vi "Get Thermal Information.vi"(8 "error in":errorcluster, 11 "All Data":T1 {"PLC Data"."PLC Data - LDO"."Timing"."Absolute Time" format="%<%H:%M:%S%3u>t"; "PLC Data"."PLC Data - LDO"."Timing"."Display Time" format="%#.20f"; "PLC Data"."PLC Data - LDO"."Timing"."Test Time Ref" format="%#.20f"; "PLC Data"."PLC Data - LDO"."Timing"."Precondition Time Ref" format="%#.20f"; "PLC Data"."PLC Data - LDO"."Timing"."First Call Time Ref" format="%#.20f"; "PLC Data"."PLC Data - FVIR"."Timing"."Absolute Time" format="%<%H:%M:%S%3u>t"; "PLC Data"."PLC Data - FVIR"."Timing"."Display Time" format="%#.20f"; "PLC Data"."PLC Data - FVIR"."Timing"."Test Time Ref" format="%#.20f"; "PLC Data"."PLC Data - FVIR"."Timing"."Precondition Time Ref" format="%#.20f"; "PLC Data"."PLC Data - FVIR"."Timing"."First Call Time Ref" format="%#.20f"}) -> (0 "error out":errorcluster, 3 "All Data Out":T1 {"PLC Data"."PLC Data - LDO"."Timing"."Absolute Time" format="%<%H:%M:%S%3u>t"; "PLC Data"."PLC Data - LDO"."Timing"."Display Time" format="%#.20f"; "PLC Data"."PLC Data - LDO"."Timing"."Test Time Ref" format="%#.20f"; "PLC Data"."PLC Data - LDO"."Timing"."Precondition Time Ref" format="%#.20f"; "PLC Data"."PLC Data - LDO"."Timing"."First Call Time Ref" format="%#.20f"; "PLC Data"."PLC Data - FVIR"."Timing"."Absolute Time" format="%<%H:%M:%S%3u>t"; "PLC Data"."PLC Data - FVIR"."Timing"."Display Time" format="%#.20f"; "PLC Data"."PLC Data - FVIR"."Timing"."Test Time Ref" format="%#.20f"; "PLC Data"."PLC Data - FVIR"."Timing"."Precondition Time Ref" format="%#.20f"; "PLC Data"."PLC Data - FVIR"."Timing"."First Call Time Ref" format="%#.20f"})   [LabVIEW 2020]
uses:
  Modbus/Modbus All Data.ctl
  Modbus/Modbus PLC Data All.ctl
  Modbus/Modbus FVIR Control.ctl
  Modbus/Modbus Timing.ctl
  <vilib>/Utility/miscctls.llb/LVDateTimeRec.ctl
  Modbus/Modbus LDO Control.ctl
  WritingDataFile/Data to Save.ctl
  Terminate Conditions Cluster.ctl
  Drivers/Inficon Transmitter/Type Definitions/Inficon Data.ctl
  Modbus/Modbus Gas Meter Data.ctl
  Drivers/Alicat LabVIEW Drivers 2v1/Sub-VIs/Data Cluster.ctl
  Drivers/Alicat LabVIEW Drivers 2v1/Sub-VIs/Units of Measure.ctl
  Gas_Rate/HEWH ANSI Rate.ctl
  Drivers/Resideo Gas Valve/Type Definitions/Vesta Info.ctl
  Thermal Calculation Cluster.ctl
panel:
  in  "LDO Full Data-Debug":string[][](array[string])=[["System Date", "06/23/2022"], ["System Time", "11:21:28.543"], ["Elapsed Time (sec)", "35"], ["PLC Real-Time Clock (Min)", "0.600000"], ["Water Inlet - Temperature (°F) - PL0001", "69.010000"], ["Water Outlet - Temperature (°F) - PL0002", "69.300000"], ["Ambient Temperature (°F)- PL0003", "68.760000"], ["Flue Exhaust Collector Box Top(°F)- PL0004", "68.970000"], ["Cold Supply Temperature (°F)- PL0005", "69.970000"], ["Hot Supply Temperature (°F)- PL0006", "68.960000"], ["TC Down (°F)- PL0007", "69.220000"], ["Ambient Temperature Outside Chamber (°F)- PL0008", "70.120000"], ["Flue Exhaust Collector Elbow (°F)- PL0009", "69.260000"], ["LDO Room Ceiling (°F)- PL0010", "69.510000"], ["Flue Gas Temperature (°F) - PL0011", "69.670000"], ["TC Type J (°F) - PL0012", "2187.000000"], ["TC Type J (°F) - PL0013", "2187.000000"], ["TC Type J (°F) - PL0014", "2187.000000"], ["TC Type K (°F) - PL0015", "2496.600000"], ["TC Type K (°F) - PL0016", "2496.600000"], ["TC Type K (°F)- PL0017", "2496.600000"], ["TC Type K (°F)- PL0018", "2496.600000"], ["Pilot Millivoltage (mV)", "0.000000"], ["Room Differential Pressure (in Water)", "0.002000"], ["Gas Manifold Pressure (in Water)", "0.120000"], ["Water Pressure Sensor (PSI)", "0.000000"], ["Flow Rate (GPM)", "0.000000"], ["Totalized Flow (Gallons)", "0.000000"], ["Counter of oil injections 0.8 cc/min", "1.000000"], ["Counter of oil injections 1.1 cc/min", "1.000000"], ["Counter of oil injections 1.33 cc/min", "13.000000"], ["Total Cycle Counter", "13.000000"], ["Absolute Pressure [inHgA]", "28.290000"], ["Gauge/Diff. Pressure [inHgG]", "-1.150000"], ["BarometricPressure [inHgA]", "29.434000"], ["Temperature [°F]", "72.800000"], ["Uncorrected [CFH]", "-0.324000"], ["Corrected [SCFH]", "-0.298000"], ["Gas Rate (BTU/hr)", "-318.821368"], ["Energy (BTU)", "0.000000"], ["Heating Value (BTU/cu.ft)", "1069.870361"], ["Totalizer [Sft3]", "0.000000"], ["Gas Selected", "NatG-1"], ["Channel Status", "Measure"], ["CO(PPMv)", "34.000"], ["CO2(%)", "0.000"], ["O2(%)", "20.890"], ["CO2 Air Free-Ultimate (%)\t\t\t\t\t\t\t\t\t", "12.200"], ["Air Free Factor", "Inf"], ["CO Air Free (%)", "Inf"], ["Water Outlet Valve-LDO", "0"], ["Water Inlet Valve-LDO", "0"], ["Gas Solenoid Valve-LDO", "1"], ["Water Flow DRK375-LDO", "0"], ["Oil Spray 0.8 cc/min-LDO", "0"], ["Oil Spray 1.1 cc/min-LDO", "0"], ["Oil Spray 1.33 cc/min-LDO", "0"], ["Heater ON/OFF-LDO", "0"], ["Water Outlet Proportional Valve-LDO", "0"], ["Conveyor ON/OFF", "0"], ["Blower ON/OFF", "0"], ["Reset LDO Totalizer (Status)", "0"]]
  # "Totalizer Timer"
  # "Totalizer Timer"
  # "Natural Gas"
  # "Propane"
  # "Totalizer Timer"
  # "Totalizer Timer"
  # "Natural Gas"
  # "Propane"
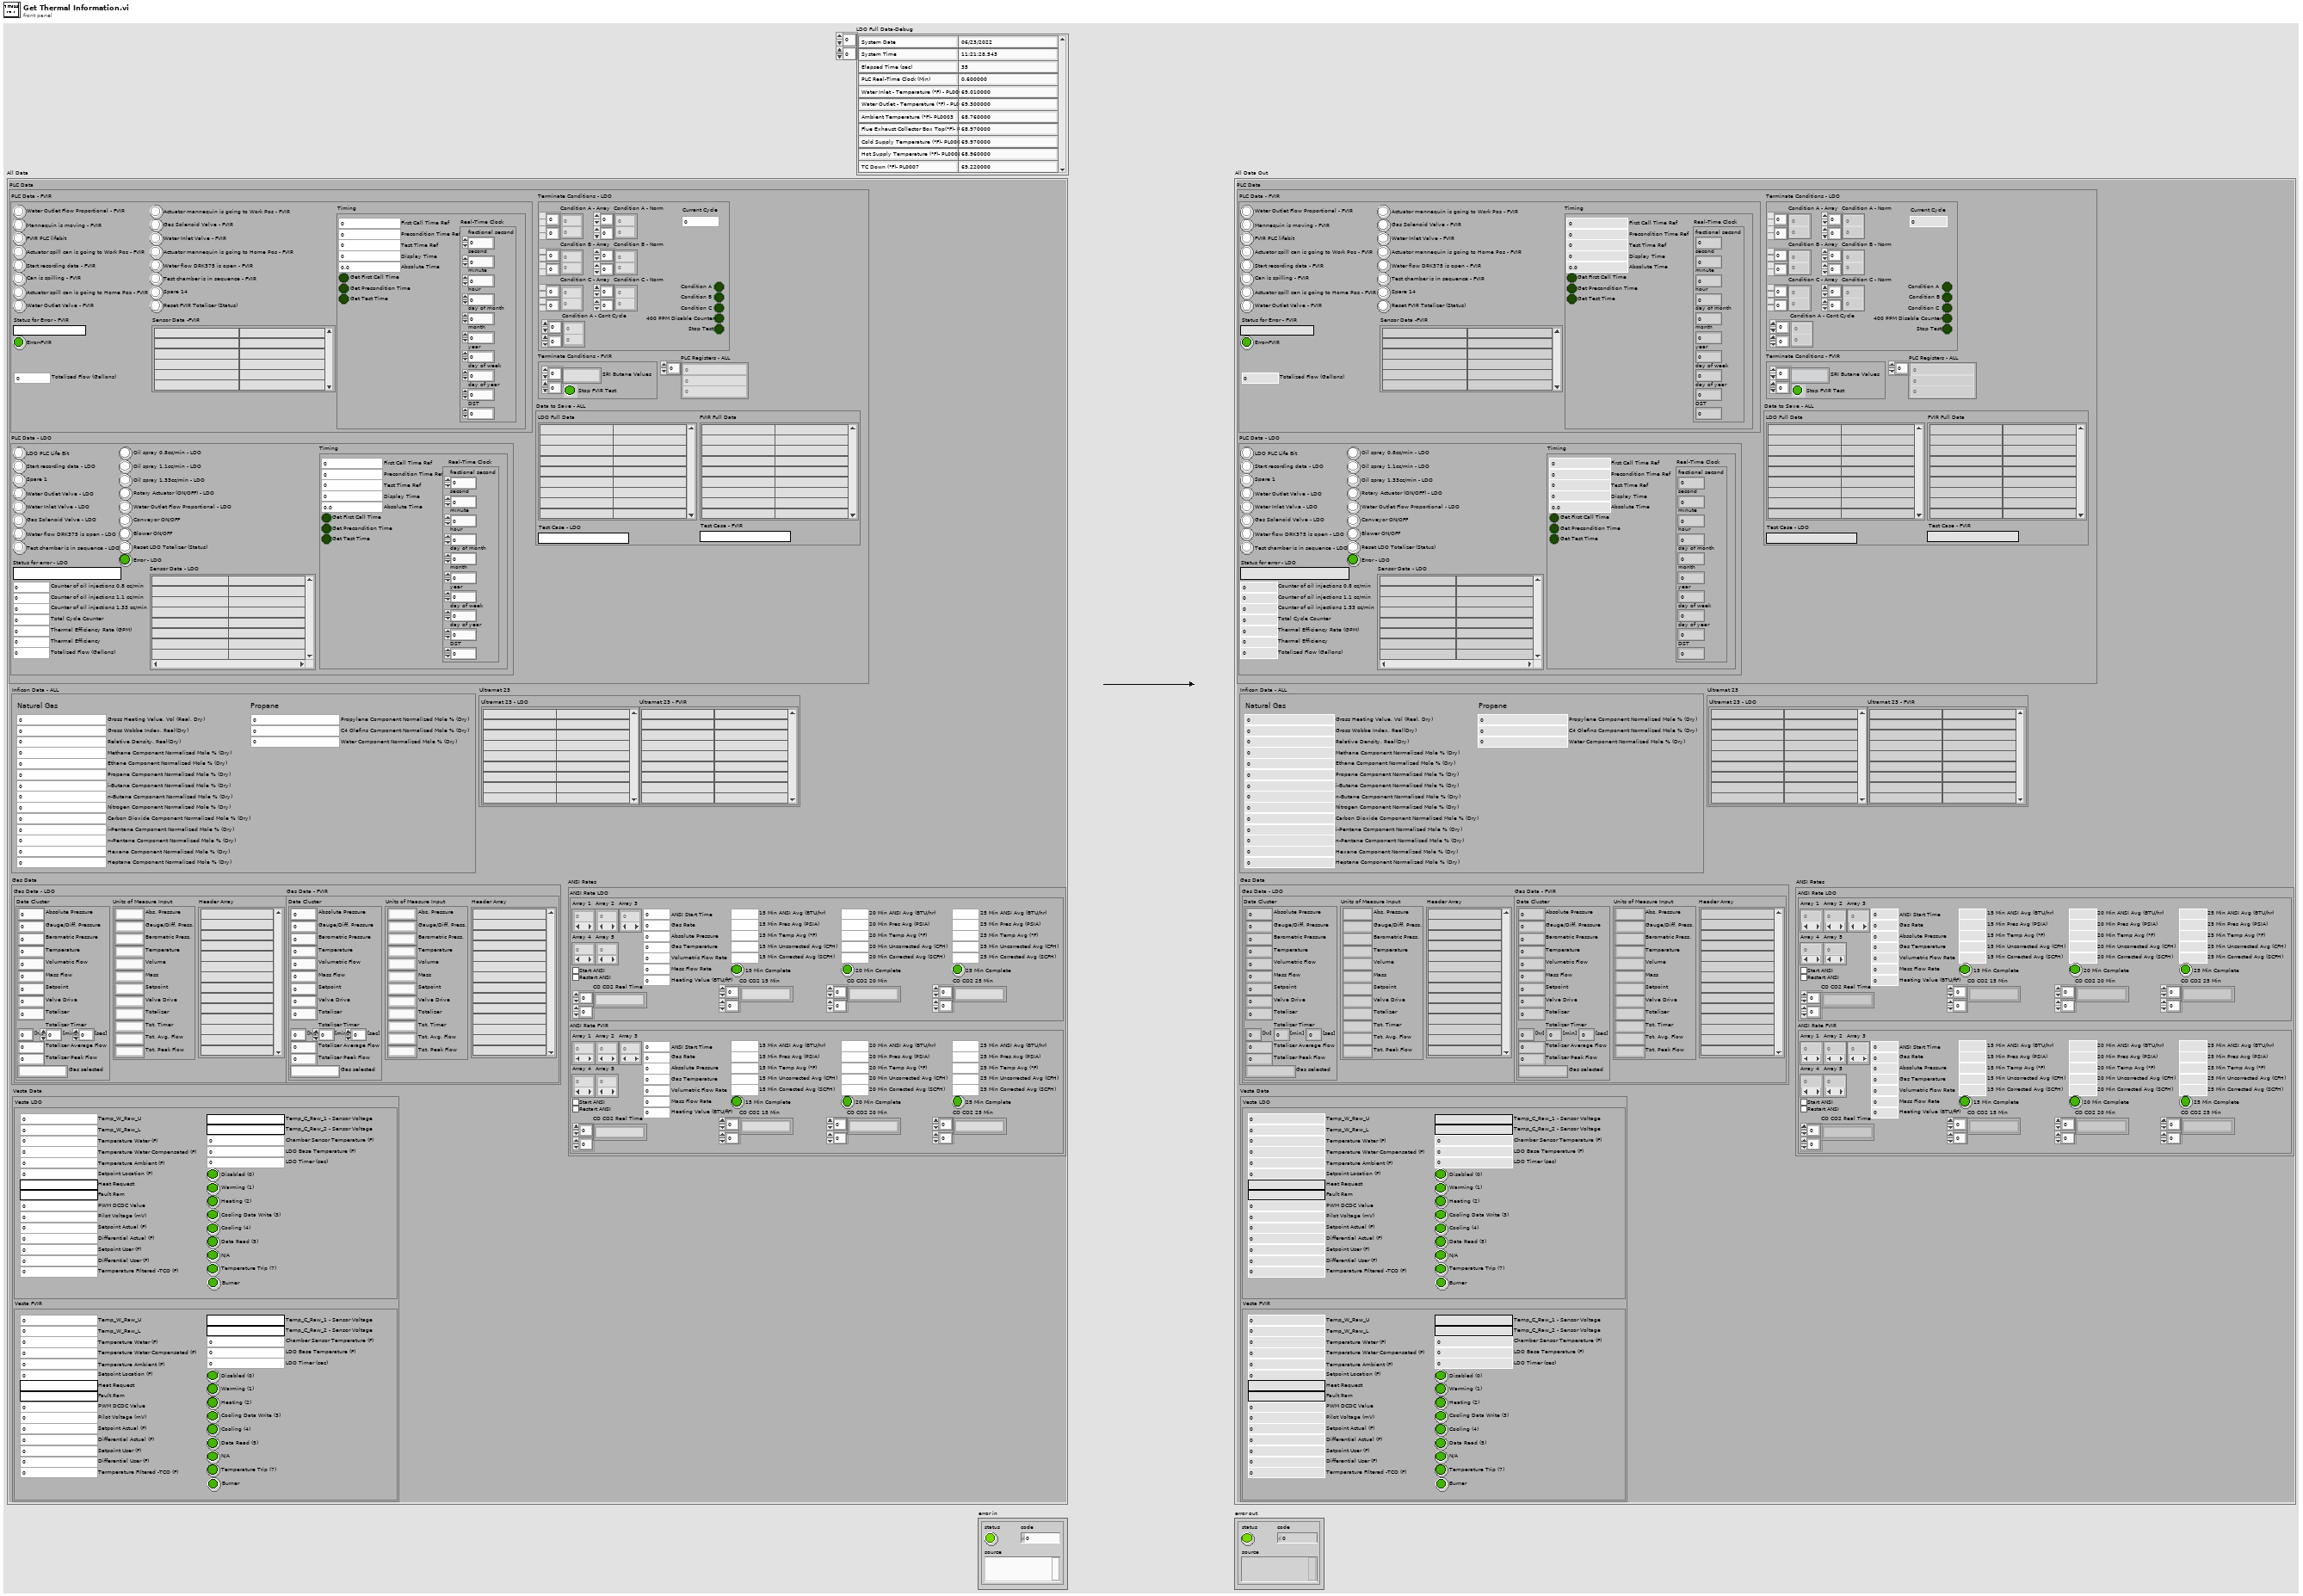
[diagram p1: front panel]
types:
  T1 = typedef "Modbus All Data.ctl" = cluster{"PLC Data":T2, "Inficon Data - ALL":T9, "Gas Data":cluster{"Gas Data - LDO":T10, "Gas Data - FVIR":T10}, "Ultramat 23":cluster{"Ultramat 23 - LDO":string[][], "Ultramat 23 - FVIR":string[][]}, "ANSI Rates":cluster{"ANSI Rate LDO":T13, "ANSI Rate FVIR":T13}, "Vesta Data":cluster{"Vesta LDO":T14, "Vesta FVIR":T14}}
  T2 = typedef "Modbus PLC Data All.ctl" = cluster{"PLC Data - FVIR":T3, "PLC Data - LDO":T6, "PLC Registers - ALL":i16[], "Data to Save - ALL":T7, "Terminate Conditions - LDO":T8, "Terminate Conditions - FVIR":cluster{"SRI Butane Values":string[][], "Stop FVIR Test":bool}}
  T3 = typedef "Modbus FVIR Control.ctl" = cluster{"Reset FVIR Totalizer (Status)":bool, "Spare 14":bool, "Actuator mannequin is going to Work Pos - FVIR":bool, "Actuator mannequin is going to Home Pos - FVIR":bool, "Test chamber is in sequence - FVIR ":bool, "Water flow DRK375 is open - FVIR":bool, "Gas Solenoid Valve - FVIR":bool, "Water Inlet Valve - FVIR":bool, "Water Outlet Flow Proportional - FVIR":bool, "Start recording data - FVIR":bool, "Actuator spill can is going to Work Pos - FVIR":bool, "Actuator spill can is going to Home Pos - FVIR":bool, "Water Outlet Valve - FVIR":bool, "Can is spilling - FVIR":bool, "Mannequin is moving - FVIR":bool, "FVIR PLC lifebit":bool, "Status for Error - FVIR":string, "Error-FVIR":bool, "Sensor Data -FVIR":string[][], "Totalized Flow (Gallons)":dbl, "Timing":T4}
  T4 = typedef "Modbus Timing.ctl" = cluster{"First Call Time Ref":dbl, "Precondition Time Ref":dbl, "Test Time Ref":dbl, "Get First Call Time":bool, "Get Precondition Time":bool, "Get Test Time":bool, "Display Time":dbl, "Real-Time Clock":T5, "Absolute Time":dbl}
  T5 = typedef "LVDateTimeRec.ctl" = cluster{"fractional second":dbl, "second":i32, "minute":i32, "hour":i32, "day of month":i32, "month":i32, "year":i32, "day of week":i32, "day of year":i32, "DST":i32}
  T6 = typedef "Modbus LDO Control.ctl" = cluster{"LDO PLC Life Bit":bool, "Start recording data - LDO":bool, "Spare 1":bool, "Water Outlet Valve - LDO":bool, "Water Inlet Valve - LDO":bool, "Gas Solenoid Valve - LDO":bool, "Water flow DRK375 is open - LDO":bool, "Test chamber is in sequence - LDO":bool, "Oil spray 0.8cc/min - LDO":bool, "Oil spray 1.1cc/min - LDO":bool, "Oil spray 1.33cc/min - LDO":bool, "Rotary Actuator (ON/OFF) - LDO":bool, "Water Outlet Flow Proportional - LDO":bool, "Conveyor ON/OFF":bool, "Blower ON/OFF":bool, "Reset LDO Totalizer (Status)":bool, "Status for error - LDO":string, "Error - LDO":bool, "Sensor Data - LDO":string[][], "Thermal Efficiency Rate (GPM)":dbl, "Thermal Efficiency":dbl, "Totalized Flow (Gallons)":dbl, "Counter of oil injections 1.33 cc/min":u16, "Total Cycle Counter":u16, "Counter of oil injections 1.1 cc/min":u16, "Counter of oil injections 0.8 cc/min":u16, "Timing":T4}
  T7 = typedef "Data to Save.ctl" = cluster{"LDO Full Data":string[][], "FVIR Full Data":string[][], "Test Case - FVIR":string, "Test Case - LDO":string}
  T8 = typedef "Terminate Conditions Cluster.ctl" = cluster{"Condition B - Array":dbl[][], "Current Cycle":u16, "Condition C - Array":dbl[][], "Condition A - Array":dbl[][], "400 PPM Disable Counter":bool, "Condition A - Norm":dbl[][], "Condition B - Norm":dbl[][], "Condition C - Norm":dbl[][], "Condition A":bool, "Condition B":bool, "Condition C":bool, "Condition A - Cont Cycle":dbl[][], "Stop Test":bool}
  T9 = typedef "Inficon Data.ctl" = cluster{"Gross Heating Value, Vol (Real, Dry)":dbl, "Nitrogen Component Normalized Mole % (Dry)":dbl, "Methane Component Normalized Mole % (Dry)":dbl, "Carbon Dioxide Component Normalized Mole % (Dry)":dbl, "Ethane Component Normalized Mole % (Dry)":dbl, "Propane Component Normalized Mole % (Dry)":dbl, "i-Pentane Component Normalized Mole % (Dry)":dbl, "i-Butane Component Normalized Mole % (Dry)":dbl, "n-Butane Component Normalized Mole % (Dry)":dbl, "n-Pentane Component Normalized Mole % (Dry)":dbl, "Hexane Component Normalized Mole % (Dry)":dbl, "Heptane Component Normalized Mole % (Dry)":dbl, "Gross Wobbe Index, Real(Dry)":dbl, "Relative Density, Real(Dry)":dbl, "Propylene Component Normalized Mole % (Dry)":dbl, "C4 Olefins Component Normalized Mole % (Dry)":dbl, "Water Component Normalized Mole % (Dry)":dbl}
  T10 = typedef "Modbus Gas Meter Data.ctl" = cluster{"Data Cluster":T11, "Units of Measure Input":T12, "Header Array":string[]}
  T11 = typedef "Data Cluster.ctl" = cluster{"Absolute Pressure":dbl, "Gauge/Diff. Pressure":dbl, "Barometric Pressure":dbl, "Temperature":dbl, "Volumetric Flow":dbl, "Mass Flow":dbl, "Setpoint":dbl, "Valve Drive":dbl, "Totalizer":dbl, "[hr]":dbl, "[min]":dbl, "[sec]":dbl, "Totalizer Average Flow":dbl, "Totalizer Peak Flow":dbl, "Gas selected":string}
  T12 = typedef "Units of Measure.ctl" = cluster{"Abs. Pressure":string, "Gauge/Diff. Press.":string, "Barometric Press.":string, "Temperature":string, "Volume":string, "Mass":string, "Setpoint":string, "Valve Drive":string, "Totalizer":string, "Tot. Timer":string, "Tot. Avg. Flow":string, "Tot. Peak Flow":string}
  T13 = typedef "HEWH ANSI Rate.ctl" = cluster{"Array 1":dbl[], "Array 3":dbl[], "Array 2":dbl[], "Start ANSI":bool, "ANSI Start Time":dbl, "Restart ANSI":bool, "15 Min ANSI Avg (BTU/hr)":dbl, "20 Min ANSI Avg (BTU/hr)":dbl, "25 Min ANSI Avg (BTU/hr)":dbl, "Absolute Pressure":dbl, "Gas Temperature":dbl, "Volumetric Flow Rate":dbl, "Mass Flow Rate":dbl, "Array 4":dbl[], "Array 5":dbl[], "Gas Rate":dbl, "15 Min Pres Avg (PSIA)":dbl, "20 Min Pres Avg (PSIA)":dbl, "25 Min Pres Avg (PSIA)":dbl, "15 Min Temp Avg (°F) ":dbl, "20 Min Temp Avg (°F)":dbl, "25 Min Temp Avg (°F)":dbl, "15 Min Uncorrected Avg (CFH)":dbl, "20 Min Uncorrected Avg (CFH)":dbl, "25 Min Uncorrected Avg (CFH)":dbl, "15 Min Corrected Avg (SCFH)":dbl, "20 Min Corrected Avg (SCFH)":dbl, "25 Min Corrected Avg (SCFH)":dbl, "15 Min Complete":bool, "20 Min Complete":bool, "25 Min Complete":bool, "Heating Value (BTU/ft³)":dbl, "CO CO2 15 Min":string[][], "CO CO2 20 Min":string[][], "CO CO2 25 Min":string[][], "CO CO2 Real Time":string[][]}
  T14 = typedef "Vesta Info.ctl" = cluster{"Temp_W_Raw_U":u16, "Temp_W_Raw_L":u16, "Temperature Water (F)":dbl, "Temperature Water Compensated (F)":dbl, "Temperature Ambient (F)":dbl, "Setpoint Location (F)":dbl, "Heat Request":string, "Fault Ram":string, "PWM DCDC Value":u16, "Pilot Voltage (mV)":dbl, "Setpoint Actual (F)":dbl, "Differential Actual (F)":dbl, "Setpoint User (F)":dbl, "Differential User (F)":dbl, "Termperature FIltered -TCO (F)":dbl, "Temp_C_Raw_1 - Sensor Voltage":string, "Temp_C_Raw_2 - Sensor Voltage":string, "Chamber Sensor Temperature (F)":dbl, "LDO Base Temperature (F)":dbl, "LDO Timer (sec)":i16, "Disabled (0)":bool, "Warming (1)":bool, "Heating (2)":bool, "Cooling Data Write (3)":bool, "Cooling (4)":bool, "Data Read (5)":bool, "N/A":bool, "Temperature Trip (7)":bool, "Burner":bool}
  T15 = typedef "Thermal Calculation Cluster.ctl" = cluster{"Gross Heating Value, Vol (Real, Dry)":dbl, "RTD Out (Deg F)":dbl, "RTD In (Deg F)":dbl, "Gallons (Gal)":dbl, "Gas Mass Flow":dbl, "Gas Totalizer":dbl, "Use Constant Thermal Efficiency":bool, "Constant Thermal Eff":dbl}
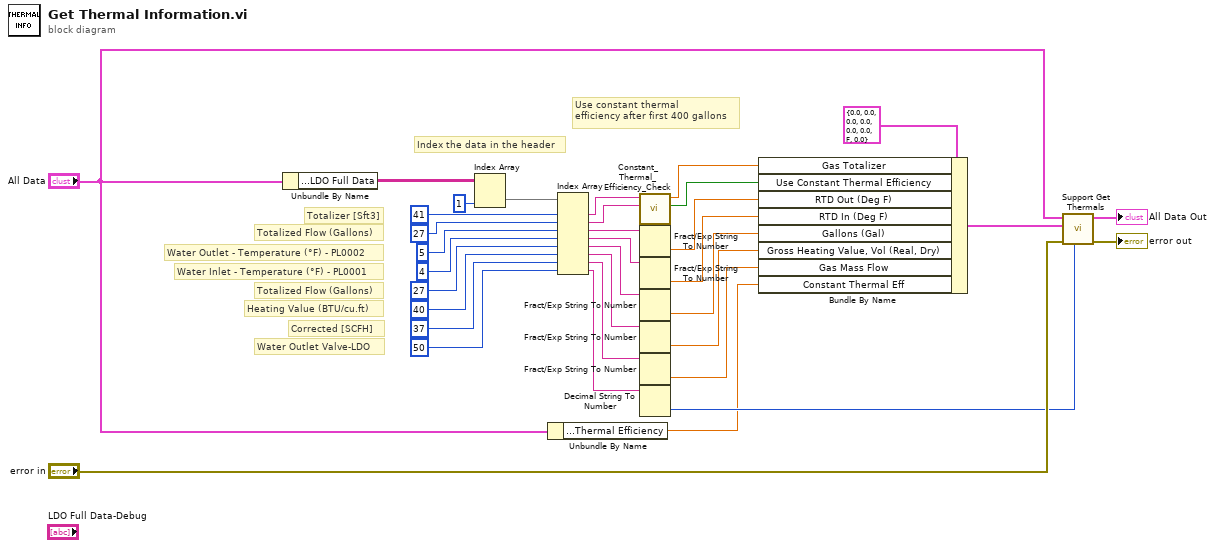
[diagram p0: block diagram]
diagram:
  # "Use constant thermal\nefficiency after first 400 gallons"
  # "Water Outlet Valve-LDO"
  # "Totalized Flow (Gallons)"
  # "Totalizer [Sft3]"
  # "Corrected [SCFH]"
  # "Heating Value (BTU/cu.ft)"
  # "Totalized Flow (Gallons)"
  # "Water Outlet - Temperature (°F) - PL0002"
  # "Water Inlet - Temperature (°F) - PL0001"
  # "Index the data in the header"
  n1 = Unbundle By Name("All Data") -> ("PLC Data.Data to Save - ALL.LDO Full Data"=w10:string[][])
  n2 = Index Array(array=w10, index (col)=1 ("disabled index (col)")) -> (element=w27:string[])  [unwired: 1 in]
  n3 = Unbundle By Name("All Data") -> ("PLC Data.PLC Data - LDO.Thermal Efficiency"=w1:dbl)
  n4 = Index Array(array=w27, index #1=41 ("index"), index #2=27 ("index"), index #3=5 ("index"), index #4=4 ("index"), index #5=27 ("index"), index #6=40 ("index"), index #7=37 ("index"), index #8=50 ("index")) -> (element #1=w26:string, element #2=w11:string, element #3=w17:string, element #4=w16:string, element #5=w15:string, element #6=w14:string, element #7=w13:string, element #8=w12:string)
  n5 = call "Constant_Thermal_Efficiency_Check.vi"("Totalized Flow (Gallons)"=w11, "Totalizer [Sft3]"=w26) -> ("Constant Thermal Efficiency?"=w7:bool, "Totalizer [Sft3]"=w8:dbl)  [unwired: 8 in]
  n6 = Fract/Exp String To Number(string=w17) -> (number=w6:dbl)  [unwired: 3 in, 1 out]
  n7 = Fract/Exp String To Number(string=w16) -> (number=w5:dbl)  [unwired: 3 in, 1 out]
  n8 = Fract/Exp String To Number(string=w15) -> (number=w4:dbl)  [unwired: 3 in, 1 out]
  n9 = Fract/Exp String To Number(string=w14) -> (number=w3:dbl)  [unwired: 3 in, 1 out]
  n10 = Fract/Exp String To Number(string=w13) -> (number=w2:dbl)  [unwired: 3 in, 1 out]
  n11 = Decimal String To Number(string=w12) -> (number=w31:i32)  [unwired: 2 in, 1 out]
  n12 = Bundle By Name(cluster=T15 {"Gross Heating Value, Vol (Real, Dry)"=0.0, "RTD Out (Deg F)"=0.0, "RTD In (Deg F)"=0.0, "Gallons (Gal)"=0.0, "Gas Mass Flow"=0.0, "Gas Totalizer"=0.0, "Use Constant Thermal Efficiency"=FALSE, "Constant Thermal Eff"=0.0} ("Input Data"), "Gas Totalizer"=w8, "Use Constant Thermal Efficiency"=w7, "RTD Out (Deg F)"=w6, "RTD In (Deg F)"=w5, "Gallons (Gal)"=w4, "Gross Heating Value, Vol (Real, Dry)"=w3, "Gas Mass Flow"=w2, "Constant Thermal Eff"=w1) -> (w29:T15)
  n13 = call "Support Get Thermals.vi"("Water Outlet Valve"=w31, "error in"="error in", "Input Data"=w29, "All Data"="All Data") -> ("error out"=→"error out":errorcluster, "All Data Out"=→"All Data Out":T1)  [unwired: 6 in]
